vi "Last Ack Creator.vi"(7 "Sender":refnum<class "Sender.lvclass">, 10 "jettl":refnum<class "jettl.lvclass">, 11 "TEMPLATE jettl in":refnum<class "TEMPLATE jettl.lvclass">) -> (3 "TEMPLATE jettl out":refnum<class "TEMPLATE jettl.lvclass">)   [LabVIEW 2021, in "_Template.lvlib" / "Templates.lvlib" / "TEMPLATE jettl.lvlib" / "TEMPLATE jettl.lvclass"]
uses:
  TEMPLATE jettl.lvclass
  TEMPLATE jettl.lvclass/TEMPLATE jettl.ctl
  jettl/jettl/jettl/jettl.lvclass
  jettl/jettl/Sender/Sender/Sender.lvclass
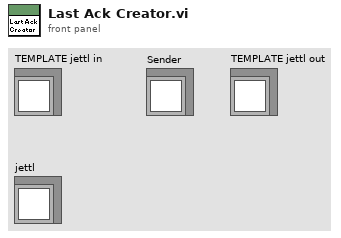
[diagram p1: front panel]
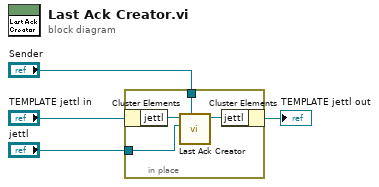
[diagram p0: block diagram]
diagram:
  n1 = in-place {
    in-place-border: "jettl" -> [w6]
    in-place-border: "Sender" -> [w5]
    n2 = in-place-cluster #1("TEMPLATE jettl in") -> ("jettl"=w8:refnum<class "jettl.lvclass">)
    n3 = call-dynamic "Last Ack Creator.vi"("Sender"=w5, "jettl"=w6, "Last Ack Creator in"=w8) -> ("Last Ack Creator out"=w7:refnum<class "jettl.lvclass">)  [unwired: 8 in]
    n4 = in-place-cluster #1("jettl"=w7) -> (→"TEMPLATE jettl out":refnum<class "TEMPLATE jettl.lvclass">)
  }
